vi "Save File DOE Extract Configuration Data.vi"(5 "Test Fixture Hardware":T2={"Power "={"Yokogawa"={"WT210"={"Sample Rate (1: 0.25s)"=1, "A Range (12: 20A)"=11, "V Range (6: 600V)"=4, "Power VISA Yokogawa WT210"=""}, "WT500"={"Power VISA Yokogawa WT500"="", "V Range (8: 1000V)"=6, "I Range (7: 40A)"=7, "Update Rate (3: 500ms)"=2}, "WT310_2"={"Sample Rate (1: 0.25s)"=1, "A Range (12: 20A)"=11, "V Range (6: 600V)"=4, "Power VISA Yokogawa WT310_2"=""}, "WT310_3"={"Sample Rate (1: 0.25s)"=1, "A Range (12: 20A)"=11, "V Range (6: 600V)"=4, "Power VISA Yokogawa WT310_3"=""}}, "Aplus"={"Aplus IP Address"="192.168.1.101", "Remote Port"=502, "Instrument"="APLUS", "Instr Driver Revision"="1.03.0053"}, "Power Limits"={"Crest Factor"={"Upper Limit"=1.49, "Lower Limit"=1.34}, "Harmonic Content"={"Uthd"=2.0}, "Voltage"={"% Error"=2.0}, "Stability"={"<1 Watt "={"Wattage"=1.0, "Slope (mW/H)"=10.0}, ">1 Watt"={"1%Power/Hour"=1.0}}}, "Nominal Voltage"=120, "Time Limit (s)"=10800.0, "Power Variation Limit (%)"=50.0, "Power Supply"={"Chroma 61605"="CHROMA", "Use Chroma?"=FALSE}}, "Weight Scale"={"Com Options"={"IND560Scale VISA"="MW100", "IP Address"="", "Remote Port"=502, "Setra Scale VISA"="SETRA", "GSE 350"="GSE350"}, "Select Scale"=""}, "Flow Rates"={"Laurel Cold IP Address"="", "Laurel Hot IP Address"="", "Hot Water Laurel VISA"="LaurelMeter_Hot", "Cold Water Laurel VISA"="LaurelMeter_Cold", "Remote Port"=0, "Laurel Communication Type"="", "Meters To Collect (Hot Cold)"="", "HOT Laurel Reference"=refnum, "COLD Laurel Reference"=refnum}, "Analog Data"={"Agilent"={"Agilent 34972_1"="34972A_1", "Agilent 34972_2"="34972A_2", "Agilent 34972_3"="34972A_3", "Agilent 34972_4"="34972A_3", "Agilent 34972_5"="34972A_3", "Agilent 34972_6"="34972A_3", "Agilent Gain"=0.0, "TC Type (K,J,T)"="", "Instrument IDN?"="", "TC Channels-List"="", "Analog Channels-List"="", "Agilent Cluster Array"=[], "TC Channels-List 2"="", "Analog Channels-List 2"=""}, "Yokogawa"={"MW100"="MW100", "Intellifaucet"=FALSE}, "Select Analog"="", "TC Coefficients"={"TC Coefficients 1"=[], "TC Coefficients 2"=[], "TC Coefficients 3"=[], "TC Coefficients 4"=[], "TC Coefficients 5"=[], "TC Coefficients 6"=[], "TC Coefficients 7"=[]}, "NI Tasks (Dryer DOE)"=["TC Temps-Module 1", "TC Temps-Module 2", "TC Temps-Module 3", "TC Temps-Module 4", "TC Temps-Module 5", "Gas and Temp-Module 6", "AC_DC Events-Module 7"], "Laurel Analog"={"Laurel IP (Water Temp)"="", "Laurel IP (Pressure)"=""}}, "ITHX-Temp Humidity"={"IP Address 1"="", "Remote Port"=0, "IP Address 2"="", "IP Address 3"=""}, "Gas Meter COM Ports"={"Gas Meter 1"="COM3", "Gas Meter 2"="COM4", "Gas Meter 3"="COM5", "Gas Meter 4"="COM6", "Gas Meter 5"="COM7", "Gas Meter 6"="COM8"}, "Barometric Pressure"={"HEISE 901A"="HEISE", "Use Barometer?"=FALSE}} {"Power"."Yokogawa"."WT310_3"."V Range (6: 600V)" items=["Auto", "15V", "30V", "60V", "150V", "300V", "600V"]; "Power"."Yokogawa"."WT310_3"."A Range (12: 20A)" items=["Auto", "5mA", "10mA", "20mA", "50mA", "100mA", "200mA", "0.5A", "1A", "2A", "5A", "10A", "20A", "50mV", "100mV", "200mV", "2.5V", "5V", "10V"]; "Power"."Yokogawa"."WT310_3"."Sample Rate (1: 0.25s)" items=["0.1s", "0.25s", "0.5s", "1s", "2s", "5s"]; "Power"."Yokogawa"."WT310_2"."V Range (6: 600V)" items=["Auto", "15V", "30V", "60V", "150V", "300V", "600V"]; "Power"."Yokogawa"."WT310_2"."A Range (12: 20A)" items=["Auto", "5mA", "10mA", "20mA", "50mA", "100mA", "200mA", "0.5A", "1A", "2A", "5A", "10A", "20A", "50mV", "100mV", "200mV", "2.5V", "5V", "10V"]; "Power"."Yokogawa"."WT310_2"."Sample Rate (1: 0.25s)" items=["0.1s", "0.25s", "0.5s", "1s", "2s", "5s"]; "Power"."Yokogawa"."WT500"."Update Rate (3: 500ms)" items=["-", "100ms", "200ms", "500ms", "1s", "2s", "5s"]; "Power"."Yokogawa"."WT500"."I Range (7: 40A)" items=["AUTO", "500 mA", "1 A", "2 A", "5 A", "10 A", "20 A", "40 A", "S-AUTO", "50 mV", "100 mV", "200 mV", "500 mV", "1 V", "2 V", "5 V", "10 V", "250 mA", "500 mA", "1 A", "2.5 A", "5 A", "10 A", "20 A", "25 mV", "50 mV", "100 mV", "250 mV", "500 mV", "1 V", "2.5 V", "5 V"]; "Power"."Yokogawa"."WT500"."V Range (8: 1000V)" items=["AUTO", "15", "30", "60", "100", "150", "300", "600", "1000", "7.5", "15", "30", "50", "75", "150", "300", "500"]; "Power"."Yokogawa"."WT210"."V Range (6: 600V)" items=["Auto", "15V", "30V", "60V", "150V", "300V", "600V"]; "Power"."Yokogawa"."WT210"."A Range (12: 20A)" items=["Auto", "5mA", "10mA", "20mA", "50mA", "100mA", "200mA", "0.5A", "1A", "2A", "5A", "10A", "20A", "50mV", "100mV", "200mV", "2.5V", "5V", "10V"]; "Power"."Yokogawa"."WT210"."Sample Rate (1: 0.25s)" items=["0.1s", "0.25s", "0.5s", "1s", "2s", "5s"]}, 7 "LV Program":T1=enum."DOE Stand", 11 "Input Config Files":string[][](array[string])) -> (1 "Drop Down Core Output":T10, 2 "Test Fixture Hardware Output":T2={"Power "={"Yokogawa"={"WT210"={"Sample Rate (1: 0.25s)"=1, "A Range (12: 20A)"=11, "V Range (6: 600V)"=4, "Power VISA Yokogawa WT210"=""}, "WT500"={"Power VISA Yokogawa WT500"="", "V Range (8: 1000V)"=6, "I Range (7: 40A)"=7, "Update Rate (3: 500ms)"=2}, "WT310_2"={"Sample Rate (1: 0.25s)"=1, "A Range (12: 20A)"=11, "V Range (6: 600V)"=4, "Power VISA Yokogawa WT310_2"=""}, "WT310_3"={"Sample Rate (1: 0.25s)"=1, "A Range (12: 20A)"=11, "V Range (6: 600V)"=4, "Power VISA Yokogawa WT310_3"=""}}, "Aplus"={"Aplus IP Address"="192.168.1.101", "Remote Port"=502, "Instrument"="APLUS", "Instr Driver Revision"="1.03.0053"}, "Power Limits"={"Crest Factor"={"Upper Limit"=1.49, "Lower Limit"=1.34}, "Harmonic Content"={"Uthd"=2.0}, "Voltage"={"% Error"=2.0}, "Stability"={"<1 Watt "={"Wattage"=1.0, "Slope (mW/H)"=10.0}, ">1 Watt"={"1%Power/Hour"=1.0}}}, "Nominal Voltage"=120, "Time Limit (s)"=10800.0, "Power Variation Limit (%)"=50.0, "Power Supply"={"Chroma 61605"="CHROMA", "Use Chroma?"=FALSE}}, "Weight Scale"={"Com Options"={"IND560Scale VISA"="MW100", "IP Address"="", "Remote Port"=502, "Setra Scale VISA"="MW100", "GSE 350"="GSE350"}, "Select Scale"=""}, "Flow Rates"={"Laurel Cold IP Address"="", "Laurel Hot IP Address"="", "Hot Water Laurel VISA"="LaurelMeter_Hot", "Cold Water Laurel VISA"="LaurelMeter_Cold", "Remote Port"=0, "Laurel Communication Type"="", "Meters To Collect (Hot Cold)"="", "HOT Laurel Reference"=refnum, "COLD Laurel Reference"=refnum}, "Analog Data"={"Agilent"={"Agilent 34972_1"="34972A_1", "Agilent 34972_2"="34972A_2", "Agilent 34972_3"="34972A_3", "Agilent 34972_4"="34972A_3", "Agilent 34972_5"="34972A_3", "Agilent 34972_6"="34972A_3", "Agilent Gain"=0.0, "TC Type (K,J,T)"="", "Instrument IDN?"="", "TC Channels-List"="", "Analog Channels-List"="", "Agilent Cluster Array"=[], "TC Channels-List 2"="", "Analog Channels-List 2"=""}, "Yokogawa"={"MW100"="MW100", "Intellifaucet"=FALSE}, "Select Analog"="", "TC Coefficients"={"TC Coefficients 1"=[], "TC Coefficients 2"=[], "TC Coefficients 3"=[], "TC Coefficients 4"=[], "TC Coefficients 5"=[], "TC Coefficients 6"=[], "TC Coefficients 7"=[]}, "NI Tasks (Dryer DOE)"=["TC Temps-Module 1", "TC Temps-Module 2", "TC Temps-Module 3", "TC Temps-Module 4", "TC Temps-Module 5", "Gas and Temp-Module 6", "AC_DC Events-Module 7"], "Laurel Analog"={"Laurel IP (Water Temp)"="", "Laurel IP (Pressure)"=""}}, "ITHX-Temp Humidity"={"IP Address 1"="", "Remote Port"=0, "IP Address 2"="", "IP Address 3"=""}, "Gas Meter COM Ports"={"Gas Meter 1"="COM3", "Gas Meter 2"="COM4", "Gas Meter 3"="COM5", "Gas Meter 4"="COM6", "Gas Meter 5"="COM7", "Gas Meter 6"="COM8"}, "Barometric Pressure"={"HEISE 901A"="HEISE", "Use Barometer?"=FALSE}} {"Power"."Yokogawa"."WT310_3"."V Range (6: 600V)" items=["Auto", "15V", "30V", "60V", "150V", "300V", "600V"]; "Power"."Yokogawa"."WT310_3"."A Range (12: 20A)" items=["Auto", "5mA", "10mA", "20mA", "50mA", "100mA", "200mA", "0.5A", "1A", "2A", "5A", "10A", "20A", "50mV", "100mV", "200mV", "2.5V", "5V", "10V"]; "Power"."Yokogawa"."WT310_3"."Sample Rate (1: 0.25s)" items=["0.1s", "0.25s", "0.5s", "1s", "2s", "5s"]; "Power"."Yokogawa"."WT310_2"."V Range (6: 600V)" items=["Auto", "15V", "30V", "60V", "150V", "300V", "600V"]; "Power"."Yokogawa"."WT310_2"."A Range (12: 20A)" items=["Auto", "5mA", "10mA", "20mA", "50mA", "100mA", "200mA", "0.5A", "1A", "2A", "5A", "10A", "20A", "50mV", "100mV", "200mV", "2.5V", "5V", "10V"]; "Power"."Yokogawa"."WT310_2"."Sample Rate (1: 0.25s)" items=["0.1s", "0.25s", "0.5s", "1s", "2s", "5s"]; "Power"."Yokogawa"."WT500"."Update Rate (3: 500ms)" items=["-", "100ms", "200ms", "500ms", "1s", "2s", "5s"]; "Power"."Yokogawa"."WT500"."I Range (7: 40A)" items=["AUTO", "500 mA", "1 A", "2 A", "5 A", "10 A", "20 A", "40 A", "S-AUTO", "50 mV", "100 mV", "200 mV", "500 mV", "1 V", "2 V", "5 V", "10 V", "250 mA", "500 mA", "1 A", "2.5 A", "5 A", "10 A", "20 A", "25 mV", "50 mV", "100 mV", "250 mV", "500 mV", "1 V", "2.5 V", "5 V"]; "Power"."Yokogawa"."WT500"."V Range (8: 1000V)" items=["AUTO", "15", "30", "60", "100", "150", "300", "600", "1000", "7.5", "15", "30", "50", "75", "150", "300", "500"]; "Power"."Yokogawa"."WT210"."V Range (6: 600V)" items=["Auto", "15V", "30V", "60V", "150V", "300V", "600V"]; "Power"."Yokogawa"."WT210"."A Range (12: 20A)" items=["Auto", "5mA", "10mA", "20mA", "50mA", "100mA", "200mA", "0.5A", "1A", "2A", "5A", "10A", "20A", "50mV", "100mV", "200mV", "2.5V", "5V", "10V"]; "Power"."Yokogawa"."WT210"."Sample Rate (1: 0.25s)" items=["0.1s", "0.25s", "0.5s", "1s", "2s", "5s"]}, 3 "Filepath Output":T8)   [LabVIEW 2016, in "File Setup.lvlib"]
uses:
  File Setup.lvlib
  File Setup (Public)/Type Definition/Save File DOE Configuration File.ctl
  File Setup (Public)/Type Definition/Save File Drop Down Controls.ctl
  File Setup (Public)/Type Definition/Save File DOE File Path Control.ctl
  File Setup (Public)/Type Definition/Save File DOE Data Save Filepaths.ctl
  Washer DOE/Type Definitions/DOE Test Fixture Hardware.ctl
  Type Definitions/UTILITY Power Inputs Control.ctl
  Drivers/IND560 Scale Monitor/Type Definitions/IND560 Configuration.ctl
  Hybrid Water Heater/Type Definitions/HEWH Agilent Cluster.ctl
  Type Definitions/UTILITY TC Coefficients.ctl
  Drivers/Omega FMA-1600A Series Gas Flow Meter/Type Definitions/FMA1600A COM Ports.ctl
  File Setup (Public)/Type Definition/Save File DOE LabView Program.ctl
panel:
  in  "Filepath":T8
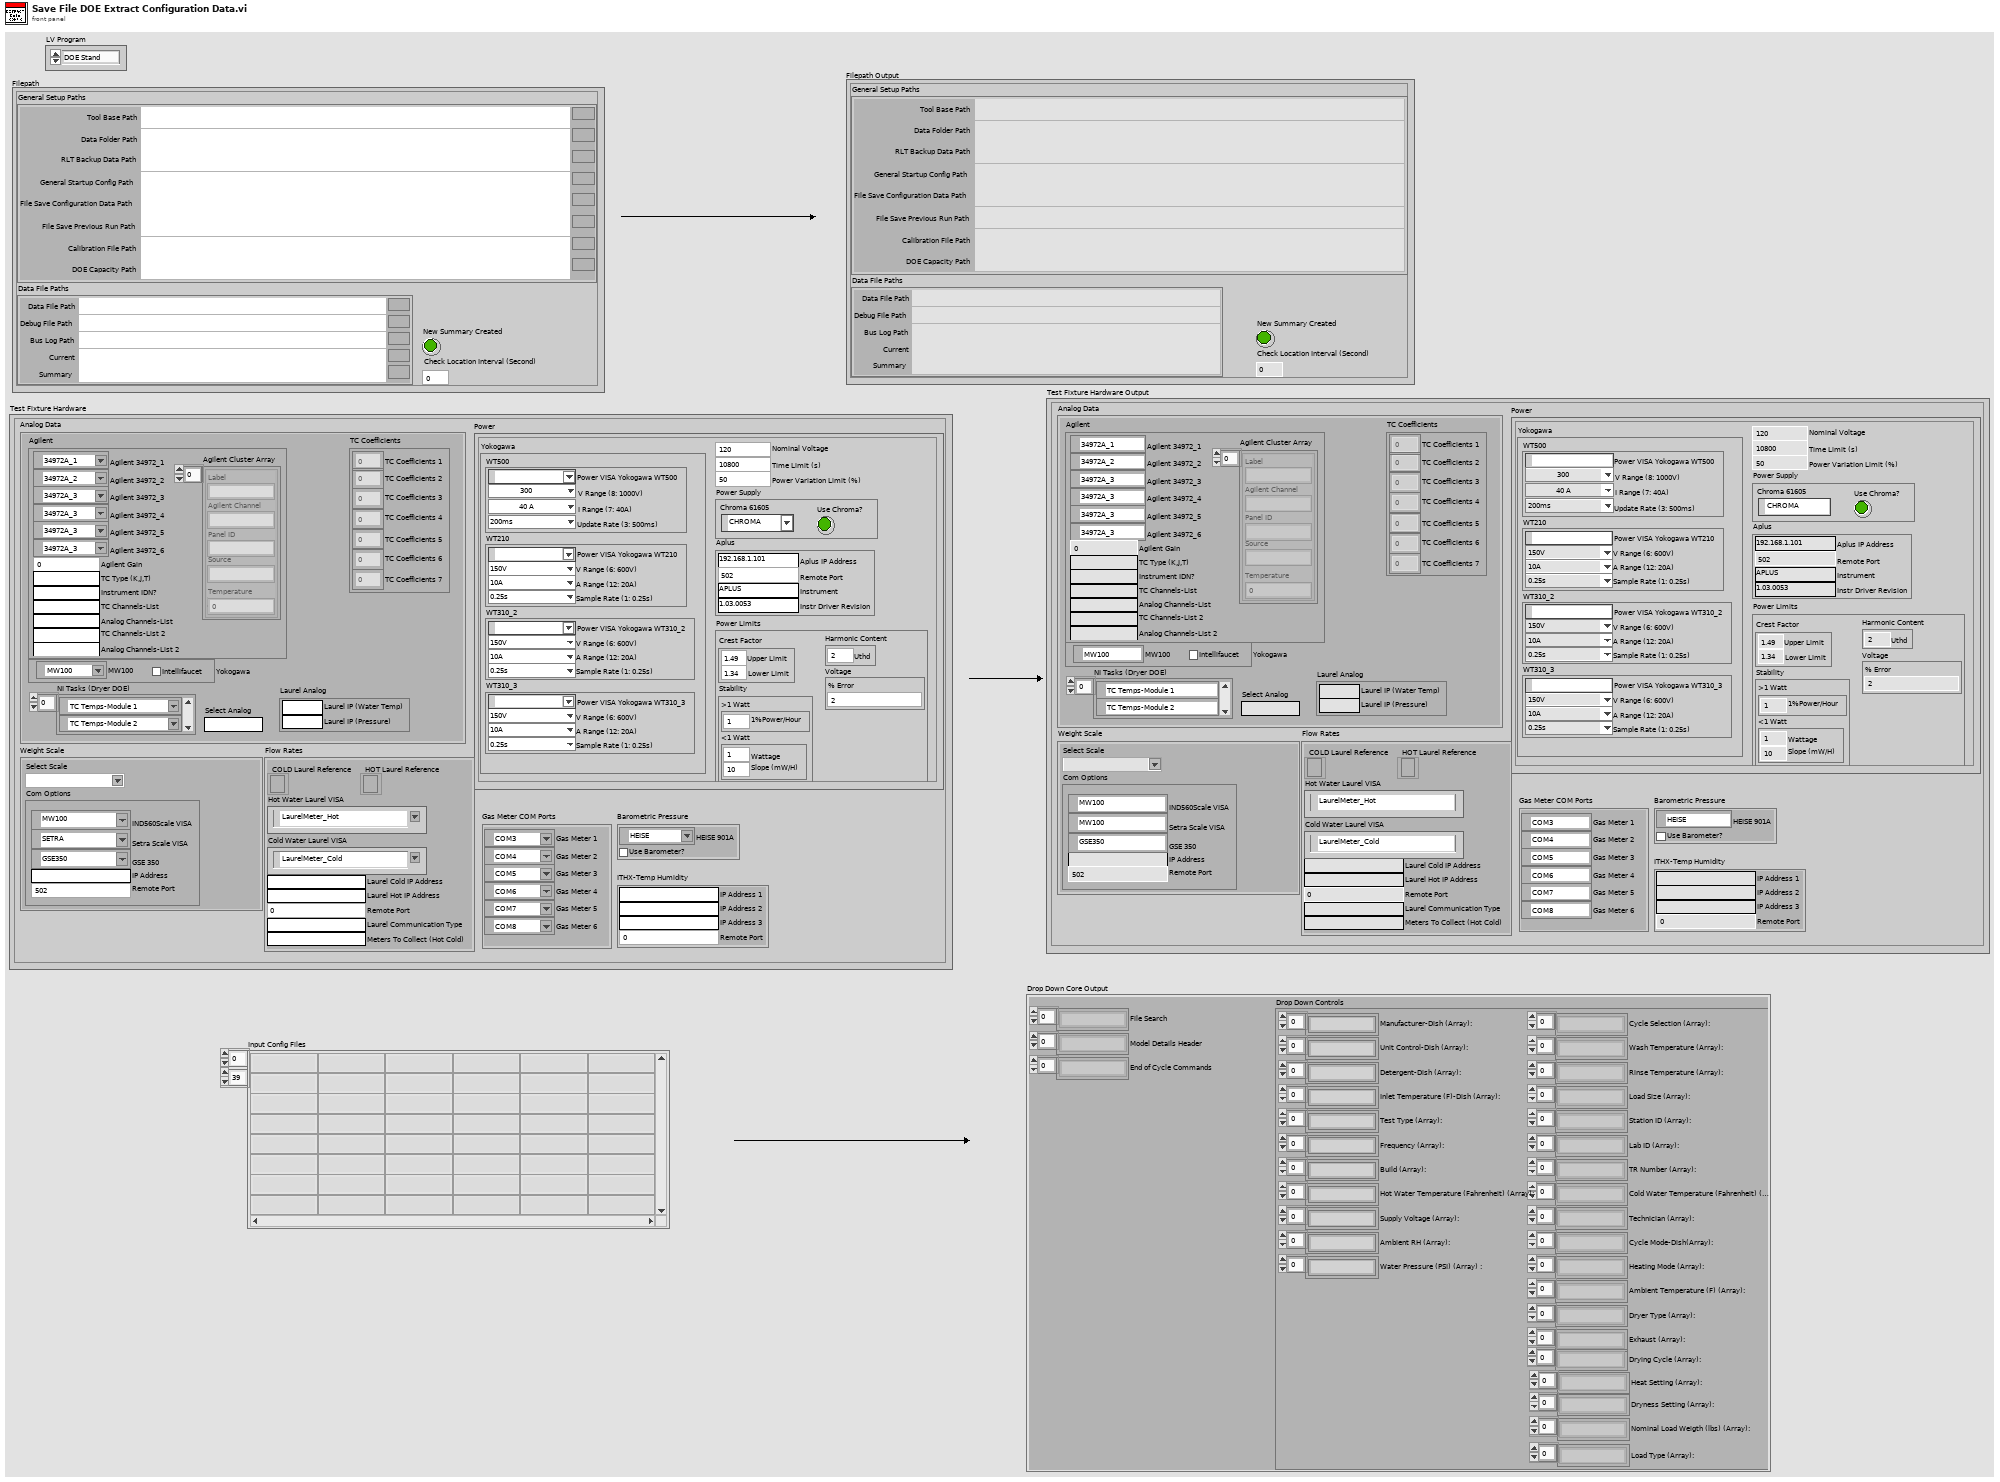
[diagram p1: front panel]
types:
  T1 = typedef "File Setup.lvlib/Save File DOE LabView Program.ctl" = enum16{"No Name Found", "DOE Stand", "Dishwasher Kitchen", "Portable Stand", "HEWH", "Dryer", "Dryer WILT", "HCC", "PRAT", "HEWH RLT", "Refrigeration"}
  T2 = typedef "DOE Test Fixture Hardware.ctl" = cluster{"Power ":T3, "Weight Scale":cluster{"Com Options":T4, "Select Scale":string}, "Flow Rates":cluster{"Laurel Cold IP Address":string, "Laurel Hot IP Address":string, "Hot Water Laurel VISA":refnum<visa-resource-name>, "Cold Water Laurel VISA":refnum<visa-resource-name>, "Remote Port":u16, "Laurel Communication Type":string, "Meters To Collect (Hot Cold)":string, "HOT Laurel Reference":refnum<k5>, "COLD Laurel Reference":refnum<k5>}, "Analog Data":cluster{"Agilent":cluster{"Agilent 34972_1":refnum<visa-resource-name>, "Agilent 34972_2":refnum<visa-resource-name>, "Agilent 34972_3":refnum<visa-resource-name>, "Agilent 34972_4":refnum<visa-resource-name>, "Agilent 34972_5":refnum<visa-resource-name>, "Agilent 34972_6":refnum<visa-resource-name>, "Agilent Gain":dbl, "TC Type (K,J,T)":string, "Instrument IDN?":string, "TC Channels-List":string, "Analog Channels-List":string, "Agilent Cluster Array":T5[], "TC Channels-List 2":string, "Analog Channels-List 2":string}, "Yokogawa":cluster{"MW100":refnum<visa-resource-name>, "Intellifaucet":bool}, "Select Analog":string, "TC Coefficients":T6, "NI Tasks (Dryer DOE)":refnum<k21>[], "Laurel Analog":cluster{"Laurel IP (Water Temp)":string, "Laurel IP (Pressure)":string}}, "ITHX-Temp Humidity":cluster{"IP Address 1":string, "Remote Port":u16, "IP Address 2":string, "IP Address 3":string}, "Gas Meter COM Ports":T7, "Barometric Pressure":cluster{"HEISE 901A":refnum<visa-resource-name>, "Use Barometer?":bool}}
  T3 = typedef "UTILITY Power Inputs Control.ctl" = cluster{"Yokogawa":cluster{"WT210":cluster{"Sample Rate (1: 0.25s)":i32, "A Range (12: 20A)":i32, "V Range (6: 600V)":i32, "Power VISA Yokogawa WT210":refnum<visa-resource-name>}, "WT500":cluster{"Power VISA Yokogawa WT500":refnum<visa-resource-name>, "V Range (8: 1000V)":i32, "I Range (7: 40A)":i32, "Update Rate (3: 500ms)":i32}, "WT310_2":cluster{"Sample Rate (1: 0.25s)":i32, "A Range (12: 20A)":i32, "V Range (6: 600V)":i32, "Power VISA Yokogawa WT310_2":refnum<visa-resource-name>}, "WT310_3":cluster{"Sample Rate (1: 0.25s)":i32, "A Range (12: 20A)":i32, "V Range (6: 600V)":i32, "Power VISA Yokogawa WT310_3":refnum<visa-resource-name>}}, "Aplus":cluster{"Aplus IP Address":string, "Remote Port":i32, "Instrument":string, "Instr Driver Revision":string}, "Power Limits":cluster{"Crest Factor":cluster{"Upper Limit":dbl, "Lower Limit":dbl}, "Harmonic Content":cluster{"Uthd":dbl}, "Voltage":cluster{"% Error":dbl}, "Stability":cluster{"<1 Watt ":cluster{"Wattage":dbl, "Slope (mW/H)":dbl}, ">1 Watt":cluster{"1%Power/Hour":dbl}}}, "Nominal Voltage":i32, "Time Limit (s)":dbl, "Power Variation Limit (%)":dbl, "Power Supply":cluster{"Chroma 61605":refnum<visa-resource-name>, "Use Chroma?":bool}}
  T4 = typedef "IND560 Configuration.ctl" = cluster{"IND560Scale VISA":refnum<visa-resource-name>, "IP Address":string, "Remote Port":u16, "Setra Scale VISA":refnum<visa-resource-name>, "GSE 350":refnum<visa-resource-name>}
  T5 = typedef "HEWH Agilent Cluster.ctl" = cluster{"Label":string, "Agilent Channel":string, "Panel ID":string, "Source":string, "Temperature":dbl}
  T6 = typedef "UTILITY TC Coefficients.ctl" = cluster{"TC Coefficients 1":dbl[], "TC Coefficients 2":dbl[], "TC Coefficients 3":dbl[], "TC Coefficients 4":dbl[], "TC Coefficients 5":dbl[], "TC Coefficients 6":dbl[], "TC Coefficients 7":dbl[]}
  T7 = typedef "FMA1600A COM Ports.ctl" = cluster{"Gas Meter 1":refnum<visa-resource-name>, "Gas Meter 2":refnum<visa-resource-name>, "Gas Meter 3":refnum<visa-resource-name>, "Gas Meter 4":refnum<visa-resource-name>, "Gas Meter 5":refnum<visa-resource-name>, "Gas Meter 6":refnum<visa-resource-name>}
  T8 = typedef "File Setup.lvlib/Save File DOE File Path Control.ctl" = cluster{"General Setup Paths":cluster{"Calibration File Path":path, "DOE Capacity Path":path, "Data Folder Path":path, "RLT Backup Data Path":path, "Tool Base Path":path, "General Startup Config Path":path, "File Save Previous Run Path":path, "File Save Configuration Data Path":path}, "Data File Paths":T9, "New Summary Created":bool, "Check Location Interval (Second)":i32}
  T9 = typedef "File Setup.lvlib/Save File DOE Data Save Filepaths.ctl" = cluster{"Data File Path":path, "Debug File Path":path, "Bus Log Path":path, "Current":path, "Summary":path}
  T10 = typedef "File Setup.lvlib/Save File DOE Configuration File.ctl" = cluster{"File Search":string[], "Model Details Header":string[], "Drop Down Controls":T11, "End of Cycle Commands":string[]}
  T11 = typedef "File Setup.lvlib/Save File Drop Down Controls.ctl" = cluster{"Manufacturer-Dish (Array):":string[], "Unit Control-Dish (Array):":string[], "Test Type (Array):":string[], "Cycle Mode-Dish(Array): ":string[], "Inlet Temperature (F)-Dish (Array):":string[], "Detergent-Dish (Array):":string[], "Cycle Selection (Array):":string[], "Wash Temperature (Array):":string[], "Rinse Temperature (Array):":string[], "Load Size (Array):":string[], "Water Pressure (PSI) (Array) :":string[], "Ambient RH (Array):":string[], "Supply Voltage (Array):":string[], "Station ID (Array):":string[], "Lab ID (Array):":string[], "TR Number (Array):":string[], "Cold Water Temperature (Fahrenheit) (Array):":string[], "Technician (Array):":string[], "Frequency (Array):":string[], "Build (Array):":string[], "Hot Water Temperature (Fahrenheit) (Array):":string[], "Heating Mode (Array):":string[], "Ambient Temperature (F) (Array):":string[], "Dryer Type (Array):":string[], "Exhaust (Array):":string[], "Drying Cycle (Array):":string[], "Heat Setting (Array):":string[], "Dryness Setting (Array):":string[], "Nominal Load Weigth (lbs) (Array):":string[], "Load Type (Array):":string[]}
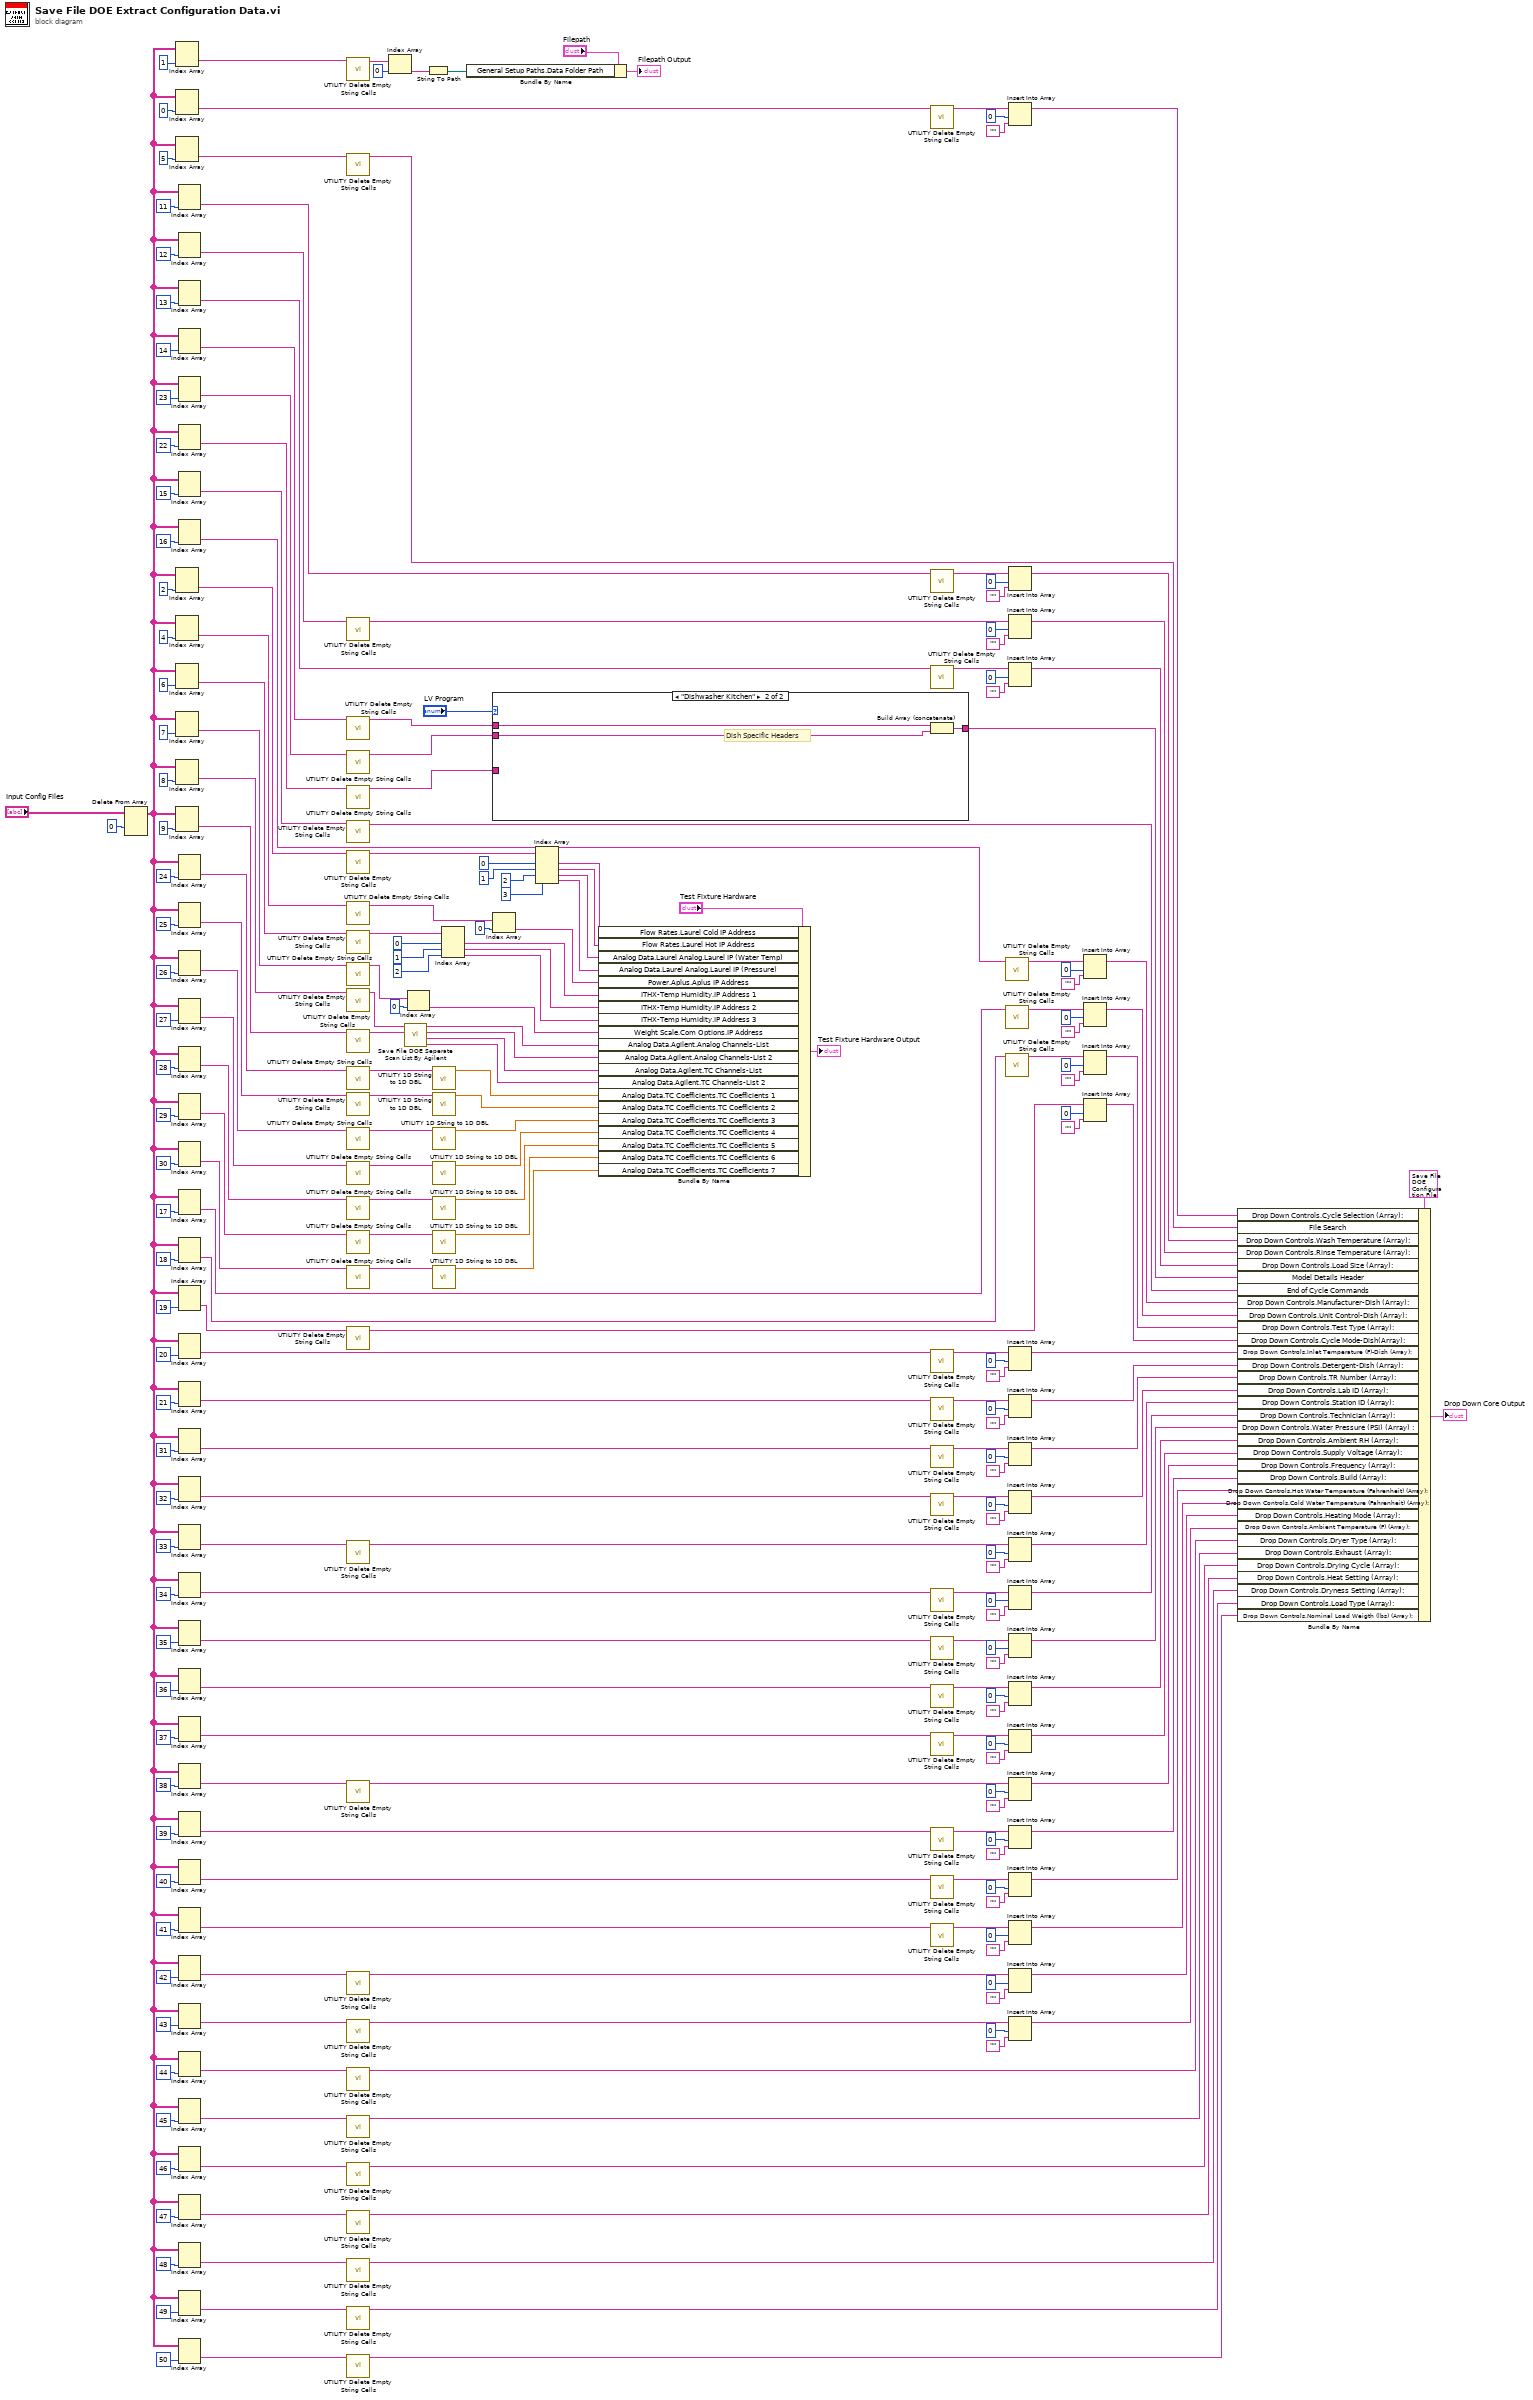
[diagram p0: block diagram]
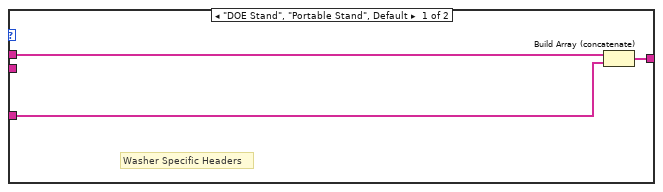
[diagram p2: hidden frame]
diagram:
  n1 = Delete From Array(array="Input Config Files", index (row)=0) -> (array with subset deleted=w22:string[][])  [unwired: 2 in, 1 out]
  n2 = Index Array(array=w22, index (col)=1 ("disabled index (col)")) -> (element=w250:string[])  [unwired: 1 in]
  n3 = Index Array(array=w22, index (col)=0 ("disabled index (col)")) -> (element=w259:string[])  [unwired: 1 in]
  n4 = Index Array(array=w22, index (col)=5 ("disabled index (col)")) -> (element=w256:string[])  [unwired: 1 in]
  n5 = Index Array(array=w22, index (col)=2 ("disabled index (col)")) -> (element=w153:string[])  [unwired: 1 in]
  n6 = Index Array(array=w22, index (col)=4 ("disabled index (col)")) -> (element=w196:string[])  [unwired: 1 in]
  n7 = Index Array(array=w22, index (col)=6 ("disabled index (col)")) -> (element=w171:string[])  [unwired: 1 in]
  n8 = Index Array(array=w22, index (col)=7 ("disabled index (col)")) -> (element=w77:string[])  [unwired: 1 in]
  n9 = Index Array(array=w22, index (col)=8 ("disabled index (col)")) -> (element=w253:string[])  [unwired: 1 in]
  n10 = Index Array(array=w22, index (col)=9 ("disabled index (col)")) -> (element=w252:string[])  [unwired: 1 in]
  n11 = Index Array(array=w22, index (col)=11 ("disabled index (col)")) -> (element=w246:string[])  [unwired: 1 in]
  n12 = Index Array(array=w22, index (col)=12 ("disabled index (col)")) -> (element=w245:string[])  [unwired: 1 in]
  n13 = Index Array(array=w22, index (col)=13 ("disabled index (col)")) -> (element=w244:string[])  [unwired: 1 in]
  n14 = Index Array(array=w22, index (col)=14 ("disabled index (col)")) -> (element=w242:string[])  [unwired: 1 in]
  n15 = Index Array(array=w22, index (col)=23 ("disabled index (col)")) -> (element=w197:string[])  [unwired: 1 in]
  n16 = Index Array(array=w22, index (col)=22 ("disabled index (col)")) -> (element=w200:string[])  [unwired: 1 in]
  n17 = Index Array(array=w22, index (col)=15 ("disabled index (col)")) -> (element=w231:string[])  [unwired: 1 in]
  n18 = Index Array(array=w22, index (col)=16 ("disabled index (col)")) -> (element=w224:string[])  [unwired: 1 in]
  n19 = Index Array(array=w22, index (col)=24 ("disabled index (col)")) -> (element=w192:string[])  [unwired: 1 in]
  n20 = Index Array(array=w22, index (col)=25 ("disabled index (col)")) -> (element=w189:string[])  [unwired: 1 in]
  n21 = Index Array(array=w22, index (col)=26 ("disabled index (col)")) -> (element=w188:string[])  [unwired: 1 in]
  n22 = Index Array(array=w22, index (col)=27 ("disabled index (col)")) -> (element=w185:string[])  [unwired: 1 in]
  n23 = Index Array(array=w22, index (col)=28 ("disabled index (col)")) -> (element=w184:string[])  [unwired: 1 in]
  n24 = Index Array(array=w22, index (col)=29 ("disabled index (col)")) -> (element=w181:string[])  [unwired: 1 in]
  n25 = Index Array(array=w22, index (col)=30 ("disabled index (col)")) -> (element=w173:string[])  [unwired: 1 in]
  n26 = Index Array(array=w22, index (col)=17 ("disabled index (col)")) -> (element=w223:string[])  [unwired: 1 in]
  n27 = Index Array(array=w22, index (col)=18 ("disabled index (col)")) -> (element=w222:string[])  [unwired: 1 in]
  n28 = Index Array(array=w22, index (col)=19 ("disabled index (col)")) -> (element=w221:string[])  [unwired: 1 in]
  n29 = Index Array(array=w22, index (col)=20 ("disabled index (col)")) -> (element=w220:string[])  [unwired: 1 in]
  n30 = Index Array(array=w22, index (col)=21 ("disabled index (col)")) -> (element=w219:string[])  [unwired: 1 in]
  n31 = Index Array(array=w22, index (col)=31 ("disabled index (col)")) -> (element=w147:string[])  [unwired: 1 in]
  n32 = Index Array(array=w22, index (col)=32 ("disabled index (col)")) -> (element=w140:string[])  [unwired: 1 in]
  n33 = Index Array(array=w22, index (col)=33 ("disabled index (col)")) -> (element=w137:string[])  [unwired: 1 in]
  n34 = Index Array(array=w22, index (col)=34 ("disabled index (col)")) -> (element=w130:string[])  [unwired: 1 in]
  n35 = Index Array(array=w22, index (col)=35 ("disabled index (col)")) -> (element=w127:string[])  [unwired: 1 in]
  n36 = Index Array(array=w22, index (col)=36 ("disabled index (col)")) -> (element=w120:string[])  [unwired: 1 in]
  n37 = Index Array(array=w22, index (col)=37 ("disabled index (col)")) -> (element=w117:string[])  [unwired: 1 in]
  n38 = Index Array(array=w22, index (col)=38 ("disabled index (col)")) -> (element=w110:string[])  [unwired: 1 in]
  n39 = Index Array(array=w22, index (col)=39 ("disabled index (col)")) -> (element=w107:string[])  [unwired: 1 in]
  n40 = Index Array(array=w22, index (col)=40 ("disabled index (col)")) -> (element=w100:string[])  [unwired: 1 in]
  n41 = Index Array(array=w22, index (col)=41 ("disabled index (col)")) -> (element=w97:string[])  [unwired: 1 in]
  n42 = Index Array(array=w22, index (col)=42 ("disabled index (col)")) -> (element=w52:string[])  [unwired: 1 in]
  n43 = Index Array(array=w22, index (col)=43 ("disabled index (col)")) -> (element=w46:string[])  [unwired: 1 in]
  n44 = Index Array(array=w22, index (col)=44 ("disabled index (col)")) -> (element=w41:string[])  [unwired: 1 in]
  n45 = Index Array(array=w22, index (col)=45 ("disabled index (col)")) -> (element=w38:string[])  [unwired: 1 in]
  n46 = Index Array(array=w22, index (col)=46 ("disabled index (col)")) -> (element=w37:string[])  [unwired: 1 in]
  n47 = Index Array(array=w22, index (col)=47 ("disabled index (col)")) -> (element=w31:string[])  [unwired: 1 in]
  n48 = Index Array(array=w22, index (col)=48 ("disabled index (col)")) -> (element=w30:string[])  [unwired: 1 in]
  n49 = Index Array(array=w22, index (col)=49 ("disabled index (col)")) -> (element=w25:string[])  [unwired: 1 in]
  n50 = Index Array(array=w22, index (col)=50 ("disabled index (col)")) -> (element=w24:string[])  [unwired: 1 in]
  n51 = call "UTILITY Delete Empty String Cells.vi"("Array with Empty Cells"=w250) -> ("Array w/o Empty Cells"=w13:string[])  [unwired: 10 in]
  n52 = call "UTILITY Delete Empty String Cells.vi"("Array with Empty Cells"=w256) -> ("Array w/o Empty Cells"=w154:string[])  [unwired: 10 in]
  n53 = call "UTILITY Delete Empty String Cells.vi"("Array with Empty Cells"=w245) -> ("Array w/o Empty Cells"=w236:string[])  [unwired: 10 in]
  n54 = call "UTILITY Delete Empty String Cells.vi"("Array with Empty Cells"=w242) -> ("Array w/o Empty Cells"=w56:string[])  [unwired: 10 in]
  n55 = call "UTILITY Delete Empty String Cells.vi"("Array with Empty Cells"=w197) -> ("Array w/o Empty Cells"=w55:string[])  [unwired: 10 in]
  n56 = call "UTILITY Delete Empty String Cells.vi"("Array with Empty Cells"=w200) -> ("Array w/o Empty Cells"=w57:string[])  [unwired: 10 in]
  n57 = call "UTILITY Delete Empty String Cells.vi"("Array with Empty Cells"=w231) -> ("Array w/o Empty Cells"=w161:string[])  [unwired: 10 in]
  n58 = call "UTILITY Delete Empty String Cells.vi"("Array with Empty Cells"=w153) -> ("Array w/o Empty Cells"=w151:string[])  [unwired: 10 in]
  n59 = call "UTILITY Delete Empty String Cells.vi"("Array with Empty Cells"=w196) -> ("Array w/o Empty Cells"=w194:string[])  [unwired: 10 in]
  n60 = call "UTILITY Delete Empty String Cells.vi"("Array with Empty Cells"=w171) -> ("Array w/o Empty Cells"=w169:string[])  [unwired: 10 in]
  n61 = call "UTILITY Delete Empty String Cells.vi"("Array with Empty Cells"=w77) -> ("Array w/o Empty Cells"=w75:string[])  [unwired: 10 in]
  n62 = call "UTILITY Delete Empty String Cells.vi"("Array with Empty Cells"=w253) -> ("Array w/o Empty Cells"=w19:string[])  [unwired: 10 in]
  n63 = call "UTILITY Delete Empty String Cells.vi"("Array with Empty Cells"=w252) -> ("Array w/o Empty Cells"=w16:string[])  [unwired: 10 in]
  n64 = call "UTILITY Delete Empty String Cells.vi"("Array with Empty Cells"=w192) -> ("Array w/o Empty Cells"=w180:string[])  [unwired: 10 in]
  n65 = call "UTILITY Delete Empty String Cells.vi"("Array with Empty Cells"=w189) -> ("Array w/o Empty Cells"=w179:string[])  [unwired: 10 in]
  n66 = call "UTILITY Delete Empty String Cells.vi"("Array with Empty Cells"=w188) -> ("Array w/o Empty Cells"=w178:string[])  [unwired: 10 in]
  n67 = call "UTILITY Delete Empty String Cells.vi"("Array with Empty Cells"=w185) -> ("Array w/o Empty Cells"=w177:string[])  [unwired: 10 in]
  n68 = call "UTILITY Delete Empty String Cells.vi"("Array with Empty Cells"=w184) -> ("Array w/o Empty Cells"=w176:string[])  [unwired: 10 in]
  n69 = call "UTILITY Delete Empty String Cells.vi"("Array with Empty Cells"=w181) -> ("Array w/o Empty Cells"=w175:string[])  [unwired: 10 in]
  n70 = call "UTILITY Delete Empty String Cells.vi"("Array with Empty Cells"=w173) -> ("Array w/o Empty Cells"=w174:string[])  [unwired: 10 in]
  n71 = call "UTILITY Delete Empty String Cells.vi"("Array with Empty Cells"=w221) -> ("Array w/o Empty Cells"=w203:string[])  [unwired: 10 in]
  n72 = call "UTILITY Delete Empty String Cells.vi"("Array with Empty Cells"=w137) -> ("Array w/o Empty Cells"=w134:string[])  [unwired: 10 in]
  n73 = call "UTILITY Delete Empty String Cells.vi"("Array with Empty Cells"=w110) -> ("Array w/o Empty Cells"=w113:string[])  [unwired: 10 in]
  n74 = call "UTILITY Delete Empty String Cells.vi"("Array with Empty Cells"=w52) -> ("Array w/o Empty Cells"=w49:string[])  [unwired: 10 in]
  n75 = call "UTILITY Delete Empty String Cells.vi"("Array with Empty Cells"=w46) -> ("Array w/o Empty Cells"=w43:string[])  [unwired: 10 in]
  n76 = call "UTILITY Delete Empty String Cells.vi"("Array with Empty Cells"=w41) -> ("Array w/o Empty Cells"=w35:string[])  [unwired: 10 in]
  n77 = call "UTILITY Delete Empty String Cells.vi"("Array with Empty Cells"=w38) -> ("Array w/o Empty Cells"=w34:string[])  [unwired: 10 in]
  n78 = call "UTILITY Delete Empty String Cells.vi"("Array with Empty Cells"=w37) -> ("Array w/o Empty Cells"=w33:string[])  [unwired: 10 in]
  n79 = call "UTILITY Delete Empty String Cells.vi"("Array with Empty Cells"=w31) -> ("Array w/o Empty Cells"=w28:string[])  [unwired: 10 in]
  n80 = call "UTILITY Delete Empty String Cells.vi"("Array with Empty Cells"=w30) -> ("Array w/o Empty Cells"=w27:string[])  [unwired: 10 in]
  n81 = call "UTILITY Delete Empty String Cells.vi"("Array with Empty Cells"=w25) -> ("Array w/o Empty Cells"=w21:string[])  [unwired: 10 in]
  n82 = call "UTILITY Delete Empty String Cells.vi"("Array with Empty Cells"=w24) -> ("Array w/o Empty Cells"=w20:string[])  [unwired: 10 in]
  n83 = Index Array(array=w13, index=0) -> (element=w11:string)
  n84 = call "Save File DOE Seperate Scan List By Agilent.vi"("TC Channel-List"=w16, "Analog Channel-List"=w19) -> ("TC List Agilent 2"=w14:string, "TC List Agilent 1"=w15:string, "Analog Channel-List 2"=w17:string, "Analog Channel-List 1"=w18:string)  [unwired: 6 in]
  n85 = Index Array(array=w75, index=0) -> (element=w70:string)
  n86 = String To Path(string=w11) -> (path=w9:path)
  n87 = call "UTILITY 1D String to 1D DBL.vi"("Save Data"=w180) -> ("DBL"=w69:dbl[])  [unwired: 10 in]
  n88 = call "UTILITY 1D String to 1D DBL.vi"("Save Data"=w179) -> ("DBL"=w68:dbl[])  [unwired: 10 in]
  n89 = call "UTILITY 1D String to 1D DBL.vi"("Save Data"=w178) -> ("DBL"=w67:dbl[])  [unwired: 10 in]
  n90 = call "UTILITY 1D String to 1D DBL.vi"("Save Data"=w177) -> ("DBL"=w66:dbl[])  [unwired: 10 in]
  n91 = call "UTILITY 1D String to 1D DBL.vi"("Save Data"=w176) -> ("DBL"=w65:dbl[])  [unwired: 10 in]
  n92 = call "UTILITY 1D String to 1D DBL.vi"("Save Data"=w175) -> ("DBL"=w64:dbl[])  [unwired: 10 in]
  n93 = call "UTILITY 1D String to 1D DBL.vi"("Save Data"=w174) -> ("DBL"=w63:dbl[])  [unwired: 10 in]
  n94 = Index Array(array=w169, index #1=0 ("index"), index #2=1 ("index"), index #3=2 ("index")) -> (element #1=w71:string, element #2=w5:string, element #3=w6:string)
  n95 = Bundle By Name(cluster="Filepath", "General Setup Paths.Data Folder Path"=w9) -> (→"Filepath Output":T8)
  n96 = case shown="\"Dishwasher Kitchen\"" "LV Program" {
    tunnel: w57 -> [w262 _]
    tunnel: w56 -> [w261 w264]
    tunnel: [w260 w263] -> w54
    tunnel: w55 -> [_ w265]
    frame "DOE Stand", "Portable Stand", Default {
      # "Washer Specific Headers"
      n97 = Build Array (concatenate)(w261, w262) -> (w260:string[])
    }
    frame "Dishwasher Kitchen" {
      # "Dish Specific Headers"
      n98 = Build Array (concatenate)(w264, w265) -> (w263:string[])
    }
  }
  n99 = Index Array(array=w194, index=0) -> (element=w72:string)
  n100 = Index Array(array=w151, index #1=0 ("index"), index #2=1 ("index"), index #3=2 ("index"), index #4=3 ("index")) -> (element #1=w74:string, element #2=w73:string, element #3=w2:string, element #4=w1:string)
  n101 = Bundle By Name(cluster="Test Fixture Hardware", "Flow Rates.Laurel Cold IP Address"=w74, "Flow Rates.Laurel Hot IP Address"=w73, "Analog Data.Laurel Analog.Laurel IP (Water Temp)"=w2, "Analog Data.Laurel Analog.Laurel IP (Pressure)"=w1, "Power.Aplus.Aplus IP Address"=w72, "ITHX-Temp Humidity.IP Address 1"=w71, "ITHX-Temp Humidity.IP Address 2"=w5, "ITHX-Temp Humidity.IP Address 3"=w6, "Weight Scale.Com Options.IP Address"=w70, "Analog Data.Agilent.Analog Channels-List"=w18, "Analog Data.Agilent.Analog Channels-List 2"=w17, "Analog Data.Agilent.TC Channels-List"=w15, "Analog Data.Agilent.TC Channels-List 2"=w14, "Analog Data.TC Coefficients.TC Coefficients 1"=w69, "Analog Data.TC Coefficients.TC Coefficients 2"=w68, "Analog Data.TC Coefficients.TC Coefficients 3"=w67, "Analog Data.TC Coefficients.TC Coefficients 4"=w66, "Analog Data.TC Coefficients.TC Coefficients 5"=w65, "Analog Data.TC Coefficients.TC Coefficients 6"=w64, "Analog Data.TC Coefficients.TC Coefficients 7"=w63) -> (→"Test Fixture Hardware Output":T2)
  n102 = call "UTILITY Delete Empty String Cells.vi"("Array with Empty Cells"=w259) -> ("Array w/o Empty Cells"=w80:string[])  [unwired: 10 in]
  n103 = call "UTILITY Delete Empty String Cells.vi"("Array with Empty Cells"=w246) -> ("Array w/o Empty Cells"=w241:string[])  [unwired: 10 in]
  n104 = call "UTILITY Delete Empty String Cells.vi"("Array with Empty Cells"=w244) -> ("Array w/o Empty Cells"=w235:string[])  [unwired: 10 in]
  n105 = call "UTILITY Delete Empty String Cells.vi"("Array with Empty Cells"=w220) -> ("Array w/o Empty Cells"=w202:string[])  [unwired: 10 in]
  n106 = call "UTILITY Delete Empty String Cells.vi"("Array with Empty Cells"=w219) -> ("Array w/o Empty Cells"=w201:string[])  [unwired: 10 in]
  n107 = call "UTILITY Delete Empty String Cells.vi"("Array with Empty Cells"=w147) -> ("Array w/o Empty Cells"=w144:string[])  [unwired: 10 in]
  n108 = call "UTILITY Delete Empty String Cells.vi"("Array with Empty Cells"=w140) -> ("Array w/o Empty Cells"=w143:string[])  [unwired: 10 in]
  n109 = call "UTILITY Delete Empty String Cells.vi"("Array with Empty Cells"=w130) -> ("Array w/o Empty Cells"=w133:string[])  [unwired: 10 in]
  n110 = call "UTILITY Delete Empty String Cells.vi"("Array with Empty Cells"=w127) -> ("Array w/o Empty Cells"=w124:string[])  [unwired: 10 in]
  n111 = call "UTILITY Delete Empty String Cells.vi"("Array with Empty Cells"=w120) -> ("Array w/o Empty Cells"=w123:string[])  [unwired: 10 in]
  n112 = call "UTILITY Delete Empty String Cells.vi"("Array with Empty Cells"=w117) -> ("Array w/o Empty Cells"=w114:string[])  [unwired: 10 in]
  n113 = call "UTILITY Delete Empty String Cells.vi"("Array with Empty Cells"=w107) -> ("Array w/o Empty Cells"=w104:string[])  [unwired: 10 in]
  n114 = call "UTILITY Delete Empty String Cells.vi"("Array with Empty Cells"=w100) -> ("Array w/o Empty Cells"=w103:string[])  [unwired: 10 in]
  n115 = call "UTILITY Delete Empty String Cells.vi"("Array with Empty Cells"=w97) -> ("Array w/o Empty Cells"=w94:string[])  [unwired: 10 in]
  n116 = call "UTILITY Delete Empty String Cells.vi"("Array with Empty Cells"=w224) -> ("Array w/o Empty Cells"=w206:string[])  [unwired: 10 in]
  n117 = call "UTILITY Delete Empty String Cells.vi"("Array with Empty Cells"=w223) -> ("Array w/o Empty Cells"=w205:string[])  [unwired: 10 in]
  n118 = call "UTILITY Delete Empty String Cells.vi"("Array with Empty Cells"=w222) -> ("Array w/o Empty Cells"=w204:string[])  [unwired: 10 in]
  n119 = Insert Into Array(array=w80, index=0, new element="") -> (w62:string[])
  n120 = Insert Into Array(array=w241, index=0, new element="") -> (w164:string[])
  n121 = Insert Into Array(array=w236, index=0, new element="") -> (w163:string[])
  n122 = Insert Into Array(array=w235, index=0, new element="") -> (w162:string[])
  n123 = Insert Into Array(array=w202, index=0, new element="") -> (w156:string[])
  n124 = Insert Into Array(array=w201, index=0, new element="") -> (w155:string[])
  n125 = Insert Into Array(array=w144, index=0, new element="") -> (w93:string[])
  n126 = Insert Into Array(array=w143, index=0, new element="") -> (w92:string[])
  n127 = Insert Into Array(array=w134, index=0, new element="") -> (w91:string[])
  n128 = Insert Into Array(array=w133, index=0, new element="") -> (w90:string[])
  n129 = Insert Into Array(array=w124, index=0, new element="") -> (w89:string[])
  n130 = Insert Into Array(array=w123, index=0, new element="") -> (w88:string[])
  n131 = Insert Into Array(array=w114, index=0, new element="") -> (w87:string[])
  n132 = Insert Into Array(array=w113, index=0, new element="") -> (w86:string[])
  n133 = Insert Into Array(array=w104, index=0, new element="") -> (w85:string[])
  n134 = Insert Into Array(array=w103, index=0, new element="") -> (w84:string[])
  n135 = Insert Into Array(array=w94, index=0, new element="") -> (w83:string[])
  n136 = Insert Into Array(array=w49, index=0, new element="") -> (w48:string[])
  n137 = Insert Into Array(array=w43, index=0, new element="") -> (w42:string[])
  n138 = Insert Into Array(array=w206, index=0, new element="") -> (w160:string[])
  n139 = Insert Into Array(array=w205, index=0, new element="") -> (w159:string[])
  n140 = Insert Into Array(array=w204, index=0, new element="") -> (w158:string[])
  n141 = Insert Into Array(array=w203, index=0, new element="") -> (w157:string[])
  n142 = Bundle By Name(cluster=T10 {"File Search"=[], "Model Details Header"=[], "Drop Down Controls"={"Manufacturer-Dish (Array):"=[], "Unit Control-Dish (Array):"=[], "Test Type (Array):"=[], "Cycle Mode-Dish(Array): "=[], "Inlet Temperature (F)-Dish (Array):"=[], "Detergent-Dish (Array):"=[], "Cycle Selection (Array):"=[], "Wash Temperature (Array):"=[], "Rinse Temperature (Array):"=[], "Load Size (Array):"=[], "Water Pressure (PSI) (Array) :"=[], "Ambient RH (Array):"=[], "Supply Voltage (Array):"=[], "Station ID (Array):"=[], "Lab ID (Array):"=[], "TR Number (Array):"=[], "Cold Water Temperature (Fahrenheit) (Array):"=[], "Technician (Array):"=[], "Frequency (Array):"=[], "Build (Array):"=[], "Hot Water Temperature (Fahrenheit) (Array):"=[], "Heating Mode (Array):"=[], "Ambient Temperature (F) (Array):"=[], "Dryer Type (Array):"=[], "Exhaust (Array):"=[], "Drying Cycle (Array):"=[], "Heat Setting (Array):"=[], "Dryness Setting (Array):"=[], "Nominal Load Weigth (lbs) (Array):"=[], "Load Type (Array):"=[]}, "End of Cycle Commands"=[]} ("input cluster"), "Drop Down Controls.Cycle Selection (Array):"=w62, "File Search"=w154, "Drop Down Controls.Wash Temperature (Array):"=w164, "Drop Down Controls.Rinse Temperature (Array):"=w163, "Drop Down Controls.Load Size (Array):"=w162, "Model Details Header"=w54, "End of Cycle Commands"=w161, "Drop Down Controls.Manufacturer-Dish (Array):"=w160, "Drop Down Controls.Unit Control-Dish (Array):"=w159, "Drop Down Controls.Test Type (Array):"=w158, "Drop Down Controls.Cycle Mode-Dish(Array):"=w157, "Drop Down Controls.Inlet Temperature (F)-Dish (Array):"=w156, "Drop Down Controls.Detergent-Dish (Array):"=w155, "Drop Down Controls.TR Number (Array):"=w93, "Drop Down Controls.Lab ID (Array):"=w92, "Drop Down Controls.Station ID (Array):"=w91, "Drop Down Controls.Technician (Array):"=w90, "Drop Down Controls.Water Pressure (PSI) (Array) :"=w89, "Drop Down Controls.Ambient RH (Array):"=w88, "Drop Down Controls.Supply Voltage (Array):"=w87, "Drop Down Controls.Frequency (Array):"=w86, "Drop Down Controls.Build (Array):"=w85, "Drop Down Controls.Hot Water Temperature (Fahrenheit) (Array):"=w84, "Drop Down Controls.Cold Water Temperature (Fahrenheit) (Array):"=w83, "Drop Down Controls.Heating Mode (Array):"=w48, "Drop Down Controls.Ambient Temperature (F) (Array):"=w42, "Drop Down Controls.Dryer Type (Array):"=w35, "Drop Down Controls.Exhaust (Array):"=w34, "Drop Down Controls.Drying Cycle (Array):"=w33, "Drop Down Controls.Heat Setting (Array):"=w28, "Drop Down Controls.Dryness Setting (Array):"=w27, "Drop Down Controls.Load Type (Array):"=w21, "Drop Down Controls.Nominal Load Weigth (lbs) (Array):"=w20) -> (→"Drop Down Core Output":T10)
